vi "Device Lib FGV.vi"(0 "Device Lib":path, 7 "Command":T1) -> (4 "Devuce Lib":path)   [LabVIEW 2013, in "Manipulate IPF.lvlib"]
uses:
  Manipulate IPF.lvlib
  type_def/Dev LIb FGV commands.ctl
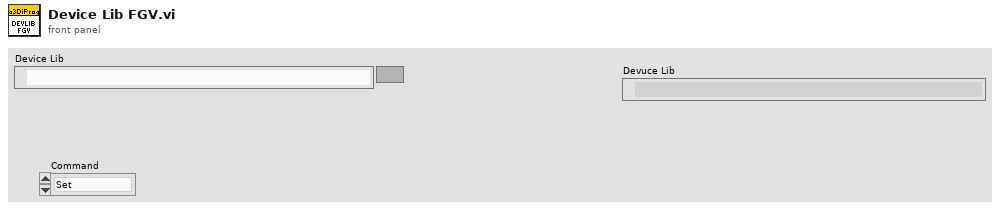
[diagram p1: front panel]
types:
  T1 = typedef "Manipulate IPF.lvlib/Dev LIb FGV commands.ctl" = enum16{"Set", "Clear", "Read"}
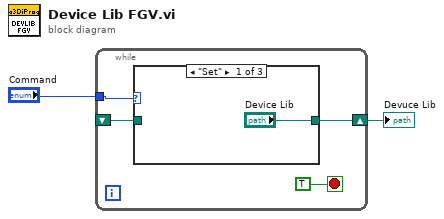
[diagram p0: block diagram]
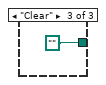
[diagram p3: hidden frame]
diagram:
  n1 = while {
    tunnel: "Command" -> [w3]
    shift-right: [w5] -> w2
    shift-left: _ -> [w4]
    stop <- TRUE stop-if-true
    n2 = case shown="\"Set\"" w3 {
      tunnel: ["Device Lib" w8 path ""] -> w5
      tunnel: w4 -> [_ w8 _]
      frame "Set" {
      }
      frame "Read" {
      }
      frame "Clear" {
      }
    }
  }
  "Devuce Lib" <- w2
